vi "Engine - Add content to Engine library.vi"(8 "error in (no error)":errorcluster, 11 "CD Wizard - Internal Data IN":T1) -> (0 "error out":errorcluster)   [LabVIEW 2015]
doc: "Add all virtual folders and VIs to the Engine library."
uses:
  TypDef/CD Wizard - Internal data.ctl
  TypDef/CD Wizard - Execution Mode.ctl
  TypDef/CD Wizard - Extra Page Name and GUID.ctl
  Constants/Constants TypDef/CD Engine lvlib.ctl
  TypDef/Add Item - Type.ctl
  Constants/CD Engine lvlib.vi
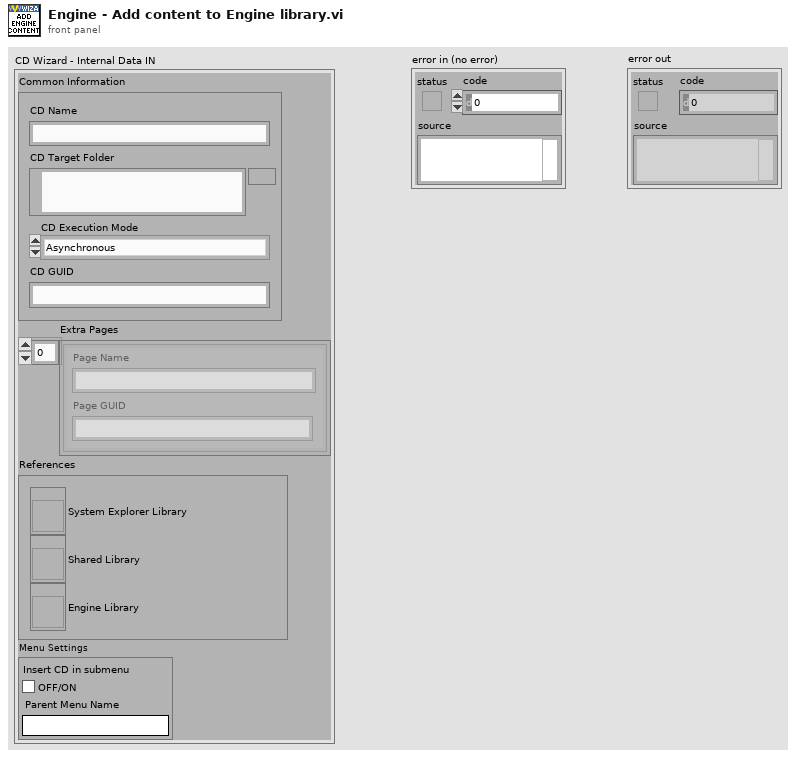
[diagram p1: front panel]
types:
  T1 = typedef "CD Wizard - Internal data.ctl" = cluster{"Common Information":cluster{"CD Name":string, "CD Target Folder":path, "CD Execution Mode":T2, "CD GUID":string}, "Extra Pages":T3[], "References":cluster{"System Explorer Library":refnum<vi>, "Shared Library":refnum<vi>, "Engine Library":refnum<vi>}, "Menu Settings":cluster{"Insert CD in submenu":bool, "Parent Menu Name":string}}
  T2 = typedef "CD Wizard - Execution Mode.ctl" = enum16{"Asynchronous", "Inline HW Interface", "Inline Model Interface", "Inline Timing and Sync", "Asynchronous Timing and Sync"}
  T3 = typedef "CD Wizard - Extra Page Name and GUID.ctl" = cluster{"Page Name":string, "Page GUID":string}
  T4 = typedef "CD Engine lvlib.ctl" = enum16{"LibraryFileName", "LibraryFolderName", "Engine.FolderName", "Engine.Init.FolderName", "Engine.Run.FolderName", "Engine.Shutdown.FolderName", "Types.FolderName", "Engine.RT Driver VI.TemplatePath", "Engine.RT Driver VI.FileName"}
  T5 = typedef "Add Item - Type.ctl" = string
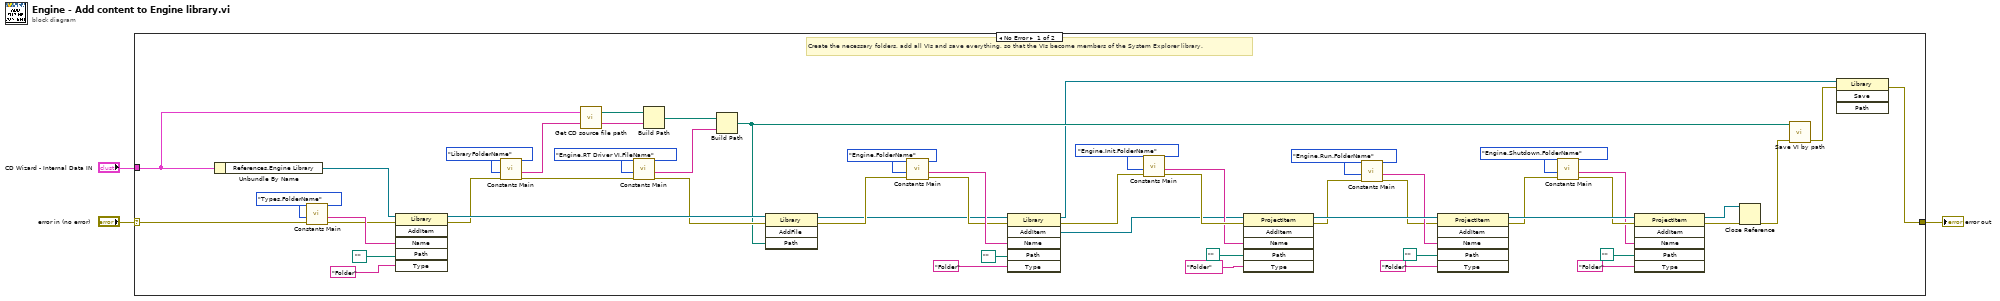
[diagram p0: block diagram]
diagram:
  n1 = case shown="No Error" "error in (no error)" {
    selector: "error in (no error)" -> [w35 w57]
    tunnel: "CD Wizard - Internal Data IN" -> [w7 _]
    tunnel: [w56 w57] -> w1
    frame No Error {
      # "Create the necessary folders, add all VIs and save everything, so that the VIs become members of the System Explorer library."
      n2 = Unbundle By Name(w7) -> ("References.Engine Library"=w34:refnum<vi>)
      n3 = call-poly "Constants Main.vi"("error in (no error)"=w35, "Action"=CD_Engine_lvlib."Types.FolderName") -> ("error out"=w51:errorcluster, "Output"=w53:string)  [unwired: 8 in]
      n4 = invoke class="Library" method="AddItem"(reference=w34, error in=w51, "Name"=w53, "Path"=path "", "Type"=T5 "Folder" ("Add Item - Type")) -> (reference out=w46:refnum<vi>, error out=w37:errorcluster)  [unwired: 1 in, 4 out]
      n5 = call-poly "Constants Main.vi"("error in (no error)"=w37, "Action"=CD_Engine_lvlib."LibraryFolderName") -> ("error out"=w43:errorcluster, "Output"=w41:string)  [unwired: 8 in]
      n6 = call "Get CD source file path.vi"("CD Wizard - Internal Data"=w7) -> ("CD Source file path"=w39:path)  [unwired: 2 in]
      n7 = call-poly "Constants Main.vi"("error in (no error)"=w43, "Action"=CD_Engine_lvlib."Engine.RT Driver VI.FileName") -> ("error out"=w36:errorcluster, "Output"=w44:string)  [unwired: 8 in]
      n8 = Build Path(base path=w39, name or relative path=w41) -> (appended path=w38:path)
      n9 = Build Path(base path=w38, name or relative path=w44) -> (appended path=w10:path)
      n10 = invoke class="Library" method="AddFile"(reference=w46, error in=w36, "Path"=w10) -> (reference out=w27:refnum<vi>, error out=w29:errorcluster)  [unwired: 1 in, 2 out]
      n11 = call-poly "Constants Main.vi"("error in (no error)"=w29, "Action"=CD_Engine_lvlib."Engine.FolderName") -> ("error out"=w28:errorcluster, "Output"=w31:string)  [unwired: 8 in]
      n12 = invoke class="Library" method="AddItem"(reference=w27, error in=w28, "Name"=w31, "Path"=path "", "Type"=T5 "Folder" ("Add Item - Type")) -> (reference out=w9:refnum<vi>, error out=w24:errorcluster, "AddItem"=w26:refnum<vi>)  [unwired: 1 in, 3 out]
      n13 = call-poly "Constants Main.vi"("error in (no error)"=w24, "Action"=CD_Engine_lvlib."Engine.Init.FolderName") -> ("error out"=w49:errorcluster, "Output"=w47:string)  [unwired: 8 in]
      n14 = invoke class="ProjectItem" method="AddItem"(reference=w26, error in=w49, "Name"=w47, "Path"=path "", "Type"=T5 "Folder" ("Add Item - Type")) -> (reference out=w23:refnum<vi>, error out=w20:errorcluster)  [unwired: 1 in, 4 out]
      n15 = call-poly "Constants Main.vi"("error in (no error)"=w20, "Action"=CD_Engine_lvlib."Engine.Run.FolderName") -> ("error out"=w17:errorcluster, "Output"=w21:string)  [unwired: 8 in]
      n16 = invoke class="ProjectItem" method="AddItem"(reference=w23, error in=w17, "Name"=w21, "Path"=path "", "Type"=T5 "Folder" ("Add Item - Type")) -> (reference out=w13:refnum<vi>, error out=w12:errorcluster)  [unwired: 1 in, 4 out]
      n17 = call-poly "Constants Main.vi"("error in (no error)"=w12, "Action"=CD_Engine_lvlib."Engine.Shutdown.FolderName") -> ("error out"=w11:errorcluster, "Output"=w8:string)  [unwired: 8 in]
      n18 = invoke class="ProjectItem" method="AddItem"(reference=w13, error in=w11, "Name"=w8, "Path"=path "", "Type"=T5 "Folder" ("Add Item - Type")) -> (reference out=w4:refnum<vi>, error out=w6:errorcluster)  [unwired: 1 in, 4 out]
      n19 = Close Reference(reference=w4, error in (no error)=w6) -> (error out=w5:errorcluster)
      n20 = call "Save VI by path.vi"("error in (no error)"=w5, "VI path"=w10) -> ("error out"=w55:errorcluster)  [unwired: 9 in]
      n21 = invoke class="Library" method="Save"(reference=w9, error in=w55) -> (error out=w56:errorcluster)  [unwired: 2 in, 3 out]
    }
    frame Error {
      # "Output default values."
    }
  }
  "error out" <- w1
